vi "Publish Cleaner.vi"(0 "Array In":T1(array[cluster])) -> (1 "Cleaned Array":T1(array[cluster]), 2 "Num Objects":u16)   [LabVIEW 2016]
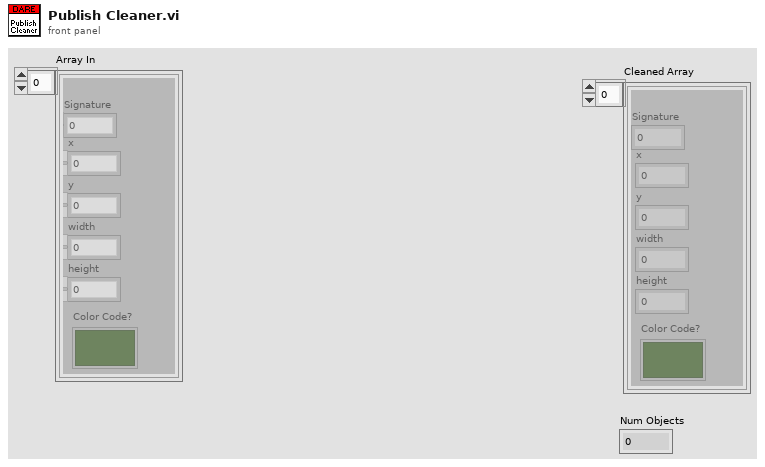
[diagram p1: front panel]
types:
  T1 = cluster{"x":u16, "y":u16, "width":u16, "height":u16, "Signature":u16, "Color Code?":bool}[]
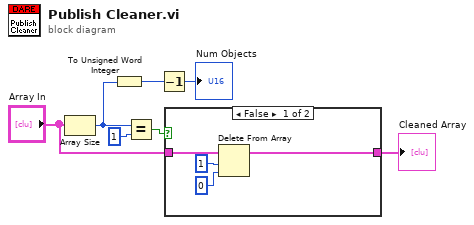
[diagram p0: block diagram]
diagram:
  n1 = Array Size(array="Array In") -> (size(s)=w3:i32)
  n2 = To Unsigned Word Integer(number=w3) -> (unsigned 16bit integer=w1:u16)
  n3 = Equal?(x=w3, y=1) -> (x = y?=w6:bool)
  n4 = Decrement(x=w1) -> (x-1=→"Num Objects":u16)
  n5 = case shown="False" w6 {
    tunnel: "Array In" -> [w11 w12]
    tunnel: [w8 w12] -> w4
    frame False {
      n6 = Delete From Array(array=w11, length=1, index=0) -> (array with subset deleted=w8:T1)  [unwired: 1 out]
    }
    frame True {
      # "If one in size, blank array."
    }
  }
  "Cleaned Array" <- w4
